vi "ConnectionReport.vi"() -> ()   [LabVIEW 2010]
panel:
  out "Connection report":string
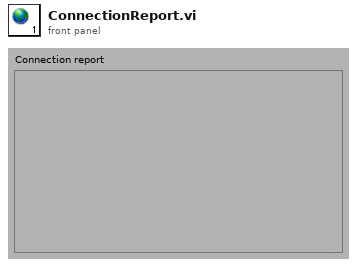
[diagram p1: front panel]
diagram:
